vi "BCU参数读取-Auto.vi"(8 "CAN端口":u16(ring), 9 "设备索引号":u16(ring), 10 "CAN卡类型":u32(ring)=21, 11 "Myindex":dbl=1.0) -> (3 "成功":bool)   [LabVIEW 2013] (continued)
                                shift-right: [w3929] -> w3923
                                shift-left: string[] [] -> [w3931]
                                i -> [w3927]
                                w3936 = 8 ("索引")
                                w3940 = 2 ("y")
                                n2325 = Multiply(x=w3927, y=w3940) -> (x*y=w3941:i32)
                                n2326 = Array Subset(array=w3942, index=w3941, length=w3940) -> (w3939:u8[])
                                n2327 = Index Array(array=w3939) -> (element #1=w3938:u8, element #2=w3937:u8)  [unwired: 2 in]
                                n2328 = call "二进制解析-8.6.vi"("索引"=w3936, "数值"=w3938) -> ("低位子数组"=w3935:i32[])  [unwired: 1 in, 2 out]
                                n2329 = call "二进制解析-8.6.vi"("索引"=w3936, "数值"=w3937) -> ("低位子数组"=w3934:i32[])  [unwired: 1 in, 2 out]
                                n2330 = Insert Into Array(array=w3935, new element=w3934) -> (w3933:i32[])  [unwired: 1 in]
                                n2331 = case shown="1" w3927 {
                                tunnel: [4 6] -> w3928
                                frame 0, Default {
                                }
                                frame 1 {
                                }
                                }
                                n2332 = Reverse 1D Array(array=w3933) -> (reversed array=w3932:i32[])
                                n2333 = for {
                                N: w3928 -> [_]
                                tunnel: w3932 -> [w3949] mode=indexing
                                tunnel: [w3945] -> w3930 mode=indexing
                                n2334 = Equal To 0?(x=w3949) -> (x = 0?=w3948:bool)
                                n2335 = Select(t="无", s=w3948, f="故障") -> (s? t:f=w3945:string)
                                }
                                n2336 = Insert Into Array(array=w3931, new element=w3930) -> (w3929:string[])  [unwired: 1 in]
                              }
                              n2337 = call "详细故障分解.vi"("名称"=string[] ["超时(pre-chg)", "后端开路(pre-chg)", "后端短路(pre-chg)", "预充电回路断开(pre-chg)", "正级继电器驱动故障(relay_driver)", "负级继电器驱动故障(relay_driver)", "预充电继电器驱动故障(relay_driver)", "充电继电器驱动故障(relay_driver)", "风机继电器驱动故障(relay_driver)", "加热继电器驱动故障(relay_driver)"], "故障输入口"=w3923) -> ("输出数组"=w3921:string[][])  [unwired: 1 in, 2 out]
                              n2338 = local write "电池故障"(w3921) -> ()
                            }
                          }
                        }
                        frame True {
                          n2339 = Index Array(array=w3953, index #1=0 ("索引"), index #2=1 ("索引")) -> (element #1=w3956:u8, element #2=w3957:u8)
                          n2340 = Join Numbers(hi=w3956, lo=w3957) -> ((hi.lo)=w3955:u16)
                          n2341 = Number To Hexadecimal String(2:w3955) -> (0:w3954:string)  [unwired: 1 out]
                          n2342 = Concatenate Strings("读取错误，代码： " ("字符串"), "0x" ("字符串"), w3954) -> (w3952:string)
                          n2343 = One Button Dialog(message=w3952, button name ("OK")="是" ("按钮名称（“确定”）")) -> ()  [unwired: 1 out]
                        }
                      }
                      n2344 = local write "消除"(FALSE ("消除")) -> ()
                      n2345 = global write "EV05全局变量1.vi" "流控帧 2"(FALSE ("流控帧 2")) -> ()
                      n2346 = local write "控制1"(FALSE ("控制1")) -> ()
                      n2347 = global write "EV05全局变量1.vi" "写入超时"(TRUE ("写入超时")) -> ()
                    }
                  }
                }
              }
            }
          }
        }
      }
      frame Error {
      }
    }
  }
  n2348 = disable-structure shown="启用" {
    disable-tunnel: w32 -> [w3968 _]
    disable-tunnel: w24 -> [w3963 _]
    disable-tunnel: w21 -> [w3962 _]
    disable-tunnel: w1 -> [w3961 _]
    frame Disabled {
      n2349 = while {
        tunnel: w3968 -> [w3977]
        tunnel: w3961 -> [w3976]
        tunnel: [w3975] -> w3967
        tunnel: [w3974] -> w3966
        tunnel: w3963 -> [_]
        tunnel: w3962 -> [_]
        stop <- w3973 stop-if-true
        n2350 = event shown="[49] \"全部读取\": 值改变" {
          selector: _ -> [_ _ _ _ _ _ _ _ _ _ _ _ _ _ _ _ _ _ _ _ _ _ _ _ _ _ _ _ _ _ _ _ _ _ _ _ _ _ _ _ _ _ _ _ _ _ _ _ _ _ _ _ _]
          dyn-events: _ -> [_ _ _ _ _ _ _ _ _ _ _ _ _ _ _ _ _ _ _ _ _ _ _ _ _ _ _ _ _ _ _ _ _ _ _ _ _ _ _ _ _ _ _ _ _ _ _ _ _ _ _ _ _]
          timeout: 200 -> [_ _ _ _ _ _ _ _ _ _ _ _ _ _ _ _ _ _ _ _ _ _ _ _ _ _ _ _ _ _ _ _ _ _ _ _ _ _ _ _ _ _ _ _ _ _ _ _ _ _ _ _ _]
          tunnel: [_ w3980 w4020 _ _ _ _ _ _ _ _ _ _ _ _ _ _ _ _ _ _ _ _ _ _ _ _ _ _ _ _ _ _ _ _ _ _ _ _ _ _ _ _ _ _ _ _ _ _ _ _ _ _] -> w3972
          tunnel: w3977 -> [w3979 w3983 w4019 _ w4060 w4071 w4082 w4093 w4098 w4109 w4120 w4131 w4142 w4153 w4170 w4181 w4197 w4735 w5157 w5182 w5210 w5313 w5386 w5398 w5408 w5454 _ _ w5504 w5571 w5638 w5705 w5772 w5839 w5906 w5974 w6042 w6109 w6176 w6246 w6257 w6296 w6318 w6358 w6380 w6418 w6478 w6513 w6549 w6582 w6651 w6684 w6717]
          tunnel: w3976 -> [w3978 w3982 w4018 _ w4059 w4070 w4081 w4092 w4097 w4108 w4119 w4130 w4141 w4152 w4169 w4180 w4196 w4734 w5156 w5181 w5209 w5312 w5384 w5396 w5407 w5453 _ _ w5503 w5570 w5637 w5704 w5771 w5838 w5905 w5973 w6041 w6108 w6175 w6244 w6256 w6295 w6317 w6357 w6379 w6417 w6477 w6512 w6548 w6581 w6650 w6683 w6716]
          tunnel: [w3979 w3983 w4019 _ w4060 w4071 w4082 w4093 w4098 w4109 w4120 w4131 w4142 w4153 w4170 w4181 w4197 w4735 w5157 w5182 w5210 w5313 w5385 w5397 w5408 w5454 _ _ w5504 w5571 w5638 w5705 w5772 w5839 w5906 w5974 w6042 w6109 w6176 w6245 w6255 w6294 w6316 w6356 w6378 w6418 w6476 w6511 w6547 w6580 w6649 w6682 w6715] -> w3975
          tunnel: [w3978 w3982 w4018 _ w4059 w4070 w4081 w4092 w4097 w4108 w4119 w4130 w4141 w4152 w4169 w4180 w4196 w4734 w5156 w5181 w5209 w5312 w5383 w5395 w5407 w5453 _ _ w5503 w5570 w5637 w5704 w5771 w5838 w5905 w5973 w6041 w6108 w6175 w6243 w6254 w6293 w6315 w6355 w6377 w6417 w6475 w6510 w6546 w6579 w6648 w6681 w6714] -> w3974
          tunnel: [_ _ _ _ _ _ _ _ _ _ _ _ _ _ _ _ _ _ _ _ _ _ _ _ _ _ _ _ _ _ _ _ _ _ _ _ _ _ _ _ w6254 w6293 w6315 w6355 w6377 _ w6475 w6510 w6546 w6579 w6648 w6681 w6714] -> w3971
          event Timeout {
            n2351 = event-data() -> ()  [unwired: 3 out]
          }
          event "停止": Value Change {
            n2352 = event-data() -> ("NewVal"=w3981:bool)  [unwired: 5 out]
            n2353 = stacked-sequence {
              tunnel: w3981 -> [w4000 _]
              tunnel: [w4000 _] -> w3980
              frame #0 {
                n2354 = global read "配置文件全局.vi" "诊断标定读取地址"() -> (w3984:path)
                n2355 = call <vilib>:"Application Directory.vi"() -> ("Application Directory"=w3994:path)
                n2356 = property class="VI"("FP.State"=T29."Hidden" ("前面板窗口:状态")) -> (reference out=w3996:refnum<vi>, error out=w3995:errorcluster)  [unwired: 2 in]
                n2357 = Build Path(base path=w3994, name or relative path="config.ini" ("名称或相对路径")) -> (appended path=w3992:path)
                n2358 = call <vilib>:"Open Config Data.vi"("configuration file path"=w3992) -> ("error out"=w3989:errorcluster, "refnum"=w3991:T25)  [unwired: 8 in, 1 out]
                n2359 = local write "停止"(TRUE ("停止")) -> ()
                n2360 = property class="VI"(reference=w3996, error in=w3995, "Front Panel.Open"=FALSE ("前面板窗口:打开")) -> ()  [unwired: 2 out]
                n2361 = call-poly <vilib>:"Write Key.vi"("section"="总信息", "error in (no error)"=w3989, "value"=w3984, "key"="诊断标定读取地址" ("section"), "refnum"=w3991) -> ("error out"=w3988:errorcluster, "refnum out"=w3987:T25)  [unwired: 4 in, 1 out]
                n2362 = call <vilib>:"Close Config Data.vi"("error in (no error)"=w3988, "refnum"=w3987) -> ("error out"=w3986:errorcluster)  [unwired: 8 in, 1 out]
                n2363 = call <vilib>:"Clear Errors.vi"("error in (no error)"=w3986) -> ()  [unwired: 6 in, 1 out]
              }
              frame #1 {
                n2364 = disable-structure shown="禁用" {
                  frame Disabled {
                    n2365 = local read "设备索引号"() -> (w4006:u16)
                    n2366 = local read "CAN卡类型"() -> (w4007:u32)
                    n2367 = local read "CAN端口"() -> (w4005:u16)
                    n2368 = Build Array(7) -> (w4002:i32[])
                    n2369 = call "transmit-8.6.vi"("can卡类型"=w4007, "设备索引号"=w4006, "CAN端口"=w4005, "ID"=418398080, "SendType"=u8 0, "Data"=w4002) -> ()  [unwired: 3 in, 11 out]
                  }
                  frame Enabled {
                    w4014 = u8 0 items=["Normal", "Listen Only"] ("工作方式")
                    w4013 = u8 1 items=["Dual Filter", "Single Filter"] ("滤波方式")
                    n2370 = local read "设备索引号"() -> (w4009:u16)
                    n2371 = local read "CAN卡类型"() -> (w4008:u32)
                    n2372 = local read "CAN端口"() -> (w4010:u16)
                    n2373 = call "CAN_Init-8.6.vi"("CAN卡类型"=w4008, "设备索引号"=w4009, "CAN端口"=w4010, "操作类型"=enum16{"初始化CAN", "关闭CAN"}."初始化CAN", "滤波方式"=w4013, "Accept Code"=u32 0, "簇"=T21 {"打开CAN"=FALSE, "初始化CAN"=TRUE, "开始CAN"=TRUE, "重启"=FALSE, "关闭CAN"=FALSE}, "Mask Code"=u32 4294967295 ("Accept Code"), "工作方式"=w4014, "是否滤波"=FALSE) -> ()  [unwired: 4 in, 6 out]
                  }
                }
              }
            }
          }
          event Panel Close? {
            n2374 = event-data() -> ()  [unwired: 5 out]
            n2375 = stacked-sequence {
              tunnel: [w4033 _] -> w4020
              frame #0 {
                w4033 = TRUE ("前面板窗口:打开")
                n2376 = global read "配置文件全局.vi" "诊断标定读取地址"() -> (w4022:path)
                n2377 = call <vilib>:"Application Directory.vi"() -> ("Application Directory"=w4032:path)
                n2378 = property class="VI"("FP.State"=T29."Hidden" ("前面板窗口:状态")) -> (reference out=w4035:refnum<vi>, error out=w4034:errorcluster)  [unwired: 2 in]
                n2379 = Build Path(base path=w4032, name or relative path="config.ini" ("名称或相对路径")) -> (appended path=w4030:path)
                n2380 = call <vilib>:"Open Config Data.vi"("configuration file path"=w4030) -> ("error out"=w4027:errorcluster, "refnum"=w4029:T25)  [unwired: 8 in, 1 out]
                n2381 = property class="VI"(reference=w4035, error in=w4034, "Front Panel.Open"=FALSE ("前面板窗口:打开")) -> ()  [unwired: 2 out]
                n2382 = call-poly <vilib>:"Write Key.vi"("section"="总信息", "error in (no error)"=w4027, "value"=w4022, "key"="诊断标定读取地址" ("section"), "refnum"=w4029) -> ("error out"=w4026:errorcluster, "refnum out"=w4025:T25)  [unwired: 4 in, 1 out]
                n2383 = call <vilib>:"Close Config Data.vi"("error in (no error)"=w4026, "refnum"=w4025) -> ("error out"=w4024:errorcluster)  [unwired: 8 in, 1 out]
                n2384 = call <vilib>:"Clear Errors.vi"("error in (no error)"=w4024) -> ()  [unwired: 6 in, 1 out]
                n2385 = local write "强制终止读写标记"(TRUE ("强制终止读写标记")) -> ()
                n2386 = local write "停止"(w4033) -> ()
              }
              frame #1 {
                w4041 = u8 0 items=["Normal", "Listen Only"] ("工作方式")
                w4042 = u8 1 items=["Dual Filter", "Single Filter"] ("滤波方式")
                n2387 = local read "设备索引号"() -> (w4046:u16)
                n2388 = local read "CAN卡类型"() -> (w4047:u32)
                n2389 = local read "CAN端口"() -> (w4045:u16)
                n2390 = call "CAN_Init-8.6.vi"("CAN卡类型"=w4047, "设备索引号"=w4046, "CAN端口"=w4045, "操作类型"=enum16{"初始化CAN", "关闭CAN"}."初始化CAN", "滤波方式"=w4042, "Accept Code"=u32 0, "簇"=T21 {"打开CAN"=FALSE, "初始化CAN"=TRUE, "开始CAN"=TRUE, "重启"=FALSE, "关闭CAN"=FALSE}, "Mask Code"=u32 4294967295 ("Accept Code"), "工作方式"=w4041, "是否滤波"=FALSE) -> ()  [unwired: 4 in, 6 out]
              }
            }
            n2391 = event-data("Discard?"=w4020) -> ()  [unwired: 1 in, 1 out]
          }
          event "终止读写按钮": Value Change {
            n2392 = event-data() -> ("NewVal"=w4048:bool)  [unwired: 6 out]
            n2393 = case shown="真" w4048 {
              frame False {
              }
              frame True {
                n2394 = local write "强制终止读写标记"(TRUE ("强制终止读写标记")) -> ()
              }
            }
          }
          event "1": Value Change {
            w4057 = FALSE ("1")
            n2395 = event-data() -> ()  [unwired: 7 out]
            n2396 = local write "主板2"(T8."项目信息" ("主从板")) -> ()
            n2397 = Not(x=w4057) -> (.not. x?=w4056:bool)
            n2398 = local write "1"(w4056) -> ()
            n2399 = local write "1 2"(w4057) -> ()
            n2400 = local write "1 3"(w4057) -> ()
            n2401 = local write "1 4"(w4057) -> ()
            n2402 = local write "1 5"(w4057) -> ()
            n2403 = local write "1 11"(w4057) -> ()
            n2404 = global read "功能码全局.vi" "主板监控2"() -> (w4055:bool[])
            n2405 = Index Array(array=w4055, index=6 ("索引")) -> (element=w4050:bool)
            n2406 = Select(t=0, s=w4050, f=1) -> (s? t:f=w4051:i32)
            n2407 = property on="项目信息" class="Tbl (严格)"("Disabled"=w4051) -> ()  [unwired: 2 in, 2 out]
            n2408 = property on="电池实际容量(A)" class="DigNum (严格)"("Disabled"=w4051) -> ()  [unwired: 2 in, 2 out]
            n2409 = property on="使用者" class="DigNum (严格)"("Disabled"=w4051) -> ()  [unwired: 2 in, 2 out]
            n2410 = property on="SOH(%)" class="DigNum (严格)"("Disabled"=w4051) -> ()  [unwired: 2 in, 2 out]
            n2411 = property on="电池额定容量(A)" class="DigNum (严格)"("Disabled"=w4051) -> ()  [unwired: 2 in, 2 out]
            n2412 = property on="SOC(%)" class="DigNum (严格)"("Disabled"=w4051) -> ()  [unwired: 2 in, 2 out]
            n2413 = property on="项目信息2" class="Clust (严格)"("DisabledEnum"=w4051) -> ()  [unwired: 2 in, 2 out]
            n2414 = property on="系统时钟" class="Str"("Disabled"=w4051) -> ()  [unwired: 2 in, 2 out]
            n2415 = property on="配置文件版本" class="Str"("Disabled"=w4051) -> ()  [unwired: 2 in, 2 out]
            n2416 = property on="车架(牌)号" class="Str"("Disabled"=w4051) -> ()  [unwired: 2 in, 2 out]
            n2417 = property on="产品编号" class="Str"("Disabled"=w4051) -> ()  [unwired: 2 in, 2 out]
          }
          event "1 2": Value Change {
            w4068 = FALSE ("1")
            n2418 = event-data() -> ()  [unwired: 7 out]
            n2419 = local write "主板2"(T8."一级故障阀值" ("主从板")) -> ()
            n2420 = Not(x=w4068) -> (.not. x?=w4067:bool)
            n2421 = local write "1"(w4068) -> ()
            n2422 = local write "1 2"(w4067) -> ()
            n2423 = local write "1 3"(w4068) -> ()
            n2424 = local write "1 4"(w4068) -> ()
            n2425 = local write "1 5"(w4068) -> ()
            n2426 = local write "1 11"(w4068) -> ()
            n2427 = global read "功能码全局.vi" "主板监控2"() -> (w4066:bool[])
            n2428 = Index Array(array=w4066, index=6 ("索引")) -> (element=w4061:bool)
            n2429 = Select(t=0, s=w4061, f=1) -> (s? t:f=w4064:i32)
            n2430 = property on="一级故障" class="Clust (严格)"("DisabledEnum"=w4064) -> ()  [unwired: 2 in, 2 out]
          }
          event "1 3": Value Change {
            w4079 = FALSE ("1")
            n2431 = event-data() -> ()  [unwired: 7 out]
            n2432 = local write "主板2"(T8."二级故障阀值" ("主从板")) -> ()
            n2433 = Not(x=w4079) -> (.not. x?=w4078:bool)
            n2434 = local write "1"(w4079) -> ()
            n2435 = local write "1 2"(w4079) -> ()
            n2436 = local write "1 3"(w4078) -> ()
            n2437 = local write "1 4"(w4079) -> ()
            n2438 = local write "1 5"(w4079) -> ()
            n2439 = local write "1 11"(w4079) -> ()
            n2440 = global read "功能码全局.vi" "主板监控2"() -> (w4077:bool[])
            n2441 = Index Array(array=w4077, index=6 ("索引")) -> (element=w4073:bool)
            n2442 = Select(t=0, s=w4073, f=1) -> (s? t:f=w4072:i32)
            n2443 = property on="一级故障 2" class="Clust (严格)"("DisabledEnum"=w4072) -> ()  [unwired: 2 in, 2 out]
          }
          event "1 4": Value Change {
            w4090 = FALSE ("1")
            n2444 = event-data() -> ()  [unwired: 7 out]
            n2445 = local write "主板2"(T8."三级故障阀值" ("主从板")) -> ()
            n2446 = Not(x=w4090) -> (.not. x?=w4089:bool)
            n2447 = local write "1"(w4090) -> ()
            n2448 = local write "1 2"(w4090) -> ()
            n2449 = local write "1 3"(w4090) -> ()
            n2450 = local write "1 4"(w4089) -> ()
            n2451 = local write "1 5"(w4090) -> ()
            n2452 = local write "1 11"(w4090) -> ()
            n2453 = global read "功能码全局.vi" "主板监控2"() -> (w4088:bool[])
            n2454 = Index Array(array=w4088, index=6 ("索引")) -> (element=w4083:bool)
            n2455 = Select(t=0, s=w4083, f=1) -> (s? t:f=w4086:i32)
            n2456 = property on="一级故障 3" class="Clust (严格)"("DisabledEnum"=w4086) -> ()  [unwired: 2 in, 2 out]
          }
          event "1 5": Value Change {
            w4095 = FALSE ("1")
            n2457 = event-data() -> ()  [unwired: 7 out]
            n2458 = local write "主板2"(T8."控制参数" ("主从板")) -> ()
            n2459 = Not(x=w4095) -> (.not. x?=w4094:bool)
            n2460 = local write "1"(w4095) -> ()
            n2461 = local write "1 2"(w4095) -> ()
            n2462 = local write "1 3"(w4095) -> ()
            n2463 = local write "1 4"(w4095) -> ()
            n2464 = local write "1 5"(w4094) -> ()
            n2465 = local write "1 11"(w4095) -> ()
            n2466 = disable-structure shown="禁用" {
              frame Disabled {
                n2467 = global read "功能码全局.vi" "主板监控2"() -> (w4102:bool[])
                n2468 = Index Array(array=w4102, index=6 ("索引")) -> (element=w4100:bool)
                n2469 = Select(t=0, s=w4100, f=1) -> (s? t:f=w4099:i32)
                n2470 = property on="风机开启温度" class="DigNum (严格)"("Disabled"=w4099) -> ()  [unwired: 2 in, 2 out]
                n2471 = property on="风机关闭温度" class="DigNum (严格)"("Disabled"=w4099) -> ()  [unwired: 2 in, 2 out]
                n2472 = property on="加热开启温度" class="DigNum (严格)"("Disabled"=w4099) -> ()  [unwired: 2 in, 2 out]
                n2473 = property on="加热关闭温度" class="DigNum (严格)"("Disabled"=w4099) -> ()  [unwired: 2 in, 2 out]
                n2474 = property on="风机开启温差" class="DigNum (严格)"("Disabled"=w4099) -> ()  [unwired: 2 in, 2 out]
                n2475 = property on="风机关闭温差" class="DigNum (严格)"("Disabled"=w4099) -> ()  [unwired: 2 in, 2 out]
                n2476 = property on="加热控制参数" class="Clust (严格)"("DisabledEnum"=w4099) -> ()  [unwired: 2 in, 2 out]
                n2477 = property on="最大允许总电压" class="DigNum (严格)"("Disabled"=w4099) -> ()  [unwired: 2 in, 2 out]
                n2478 = property on="最大允许充电温度" class="DigNum (严格)"("Disabled"=w4099) -> ()  [unwired: 2 in, 2 out]
                n2479 = property on="最小允许充电温度" class="DigNum (严格)"("Disabled"=w4099) -> ()  [unwired: 2 in, 2 out]
                n2480 = property on="电流步长" class="DigNum (严格)"("Disabled"=w4099) -> ()  [unwired: 2 in, 2 out]
                n2481 = property on="最大允许单体电压" class="DigNum (严格)"("Disabled"=w4099) -> ()  [unwired: 2 in, 2 out]
                n2482 = property on="最小允许单体电压" class="DigNum (严格)"("Disabled"=w4099) -> ()  [unwired: 2 in, 2 out]
                n2483 = property on="最大允许充电电流" class="DigNum (严格)"("Disabled"=w4099) -> ()  [unwired: 2 in, 2 out]
                n2484 = property on="最小允许充电电流" class="DigNum (严格)"("Disabled"=w4099) -> ()  [unwired: 2 in, 2 out]
              }
              frame Enabled {
              }
            }
          }
          event "1 11": Value Change {
            w4106 = FALSE ("1")
            n2485 = event-data() -> ()  [unwired: 7 out]
            n2486 = local write "主板2"(T8."电池信息" ("主从板")) -> ()
            n2487 = Not(x=w4106) -> (.not. x?=w4105:bool)
            n2488 = local write "1"(w4106) -> ()
            n2489 = local write "1 2"(w4106) -> ()
            n2490 = local write "1 3"(w4106) -> ()
            n2491 = local write "1 4"(w4106) -> ()
            n2492 = local write "1 5"(w4106) -> ()
            n2493 = local write "1 11"(w4105) -> ()
            n2494 = disable-structure shown="禁用" {
              frame Disabled {
                n2495 = global read "功能码全局.vi" "主板监控2"() -> (w4112:bool[])
                n2496 = Index Array(array=w4112, index=6 ("索引")) -> (element=w4110:bool)
                n2497 = Select(t=0, s=w4110, f=1) -> (s? t:f=w4113:i32)
                n2498 = property on="电池串联" class="DigNum (严格)"("Disabled"=w4113) -> ()  [unwired: 2 in, 2 out]
                n2499 = property on="电池并联" class="DigNum (严格)"("Disabled"=w4113) -> ()  [unwired: 2 in, 2 out]
                n2500 = property on="电池包额定容量" class="DigNum (严格)"("Disabled"=w4113) -> ()  [unwired: 2 in, 2 out]
                n2501 = property on="电池包额定能量(kWh)" class="DigNum (严格)"("Disabled"=w4113) -> ()  [unwired: 2 in, 2 out]
                n2502 = property on="电池包额定总电压" class="DigNum (严格)"("Disabled"=w4113) -> ()  [unwired: 2 in, 2 out]
                n2503 = property on="实际容量" class="DigNum (严格)"("Disabled"=w4113) -> ()  [unwired: 2 in, 2 out]
                n2504 = property on="电池包组号" class="Str"("Disabled"=w4113) -> ()  [unwired: 2 in, 2 out]
                n2505 = property on="电池生产日期" class="Str"("Disabled"=w4113) -> ()  [unwired: 2 in, 2 out]
                n2506 = property on="电池厂家" class="Str"("Disabled"=w4113) -> ()  [unwired: 2 in, 2 out]
                n2507 = property on="电池类型" class="Str"("Disabled"=w4113) -> ()  [unwired: 2 in, 2 out]
                n2508 = property on="累计充电总安时" class="DigNum (严格)"("Disabled"=w4113) -> ()  [unwired: 2 in, 2 out]
                n2509 = property on="累计放电总安时" class="DigNum (严格)"("Disabled"=w4113) -> ()  [unwired: 2 in, 2 out]
                n2510 = property on="电池放空次数" class="DigNum (严格)"("Disabled"=w4113) -> ()  [unwired: 2 in, 2 out]
                n2511 = property on="电池充满次数" class="DigNum (严格)"("Disabled"=w4113) -> ()  [unwired: 2 in, 2 out]
                n2512 = property on="电池充电次数" class="DigNum (严格)"("Disabled"=w4113) -> ()  [unwired: 2 in, 2 out]
                n2513 = property on="电池信息" class="Clust (严格)"("DisabledEnum"=w4113) -> ()  [unwired: 2 in, 2 out]
              }
              frame Enabled {
              }
            }
          }
          event "1 6": Value Change {
            w4117 = FALSE ("1 6")
            n2514 = event-data() -> ()  [unwired: 7 out]
            n2515 = Not(x=w4117) -> (.not. x?=w4116:bool)
            n2516 = local write "1 6"(w4116) -> ()
            n2517 = local write "1 7"(w4117) -> ()
            n2518 = local write "1 8"(w4117) -> ()
            n2519 = local write "1 9"(w4117) -> ()
            n2520 = local write "1 10"(w4117) -> ()
            n2521 = local write "等级 2"(T19."从板信息" ("等级 2")) -> ()
            n2522 = disable-structure shown="禁用" {
              frame Disabled {
                n2523 = global read "功能码全局.vi" "主板监控2"() -> (w4123:bool[])
                n2524 = Index Array(array=w4123, index=6 ("索引")) -> (element=w4121:bool)
                n2525 = Select(t=0, s=w4121, f=1) -> (s? t:f=w4124:i32)
                n2526 = property on="项目信息 2" class="Tbl (严格)"("Disabled"=w4124) -> ()  [unwired: 2 in, 2 out]
                n2527 = property on="加热控制参数" class="Clust (严格)"("Disabled"=w4124) -> ()  [unwired: 2 in, 2 out]
              }
              frame Enabled {
              }
            }
          }
          event "1 7": Value Change {
            w4128 = FALSE ("1 6")
            n2528 = event-data() -> ()  [unwired: 7 out]
            n2529 = disable-structure shown="禁用" {
              frame Disabled {
                n2530 = global read "功能码全局.vi" "主板监控2"() -> (w4137:bool[])
                n2531 = Index Array(array=w4137, index=6 ("索引")) -> (element=w4132:bool)
                n2532 = Select(t=0, s=w4132, f=1) -> (s? t:f=w4133:i32)
                n2533 = property on="一级故障 6" class="Clust (严格)"("DisabledEnum"=w4133) -> ()  [unwired: 2 in, 2 out]
              }
              frame Enabled {
              }
            }
            n2534 = local write "等级 2"(T19."一级故障阀值" ("等级 2")) -> ()
            n2535 = Not(x=w4128) -> (.not. x?=w4127:bool)
            n2536 = local write "1 6"(w4128) -> ()
            n2537 = local write "1 7"(w4127) -> ()
            n2538 = local write "1 8"(w4128) -> ()
            n2539 = local write "1 9"(w4128) -> ()
            n2540 = local write "1 10"(w4128) -> ()
          }
          event "1 8": Value Change {
            w4139 = FALSE ("1 6")
            n2541 = event-data() -> ()  [unwired: 7 out]
            n2542 = disable-structure shown="禁用" {
              frame Disabled {
                n2543 = global read "功能码全局.vi" "主板监控2"() -> (w4148:bool[])
                n2544 = Index Array(array=w4148, index=6 ("索引")) -> (element=w4143:bool)
                n2545 = Select(t=0, s=w4143, f=1) -> (s? t:f=w4144:i32)
                n2546 = property on="一级故障 7" class="Clust (严格)"("DisabledEnum"=w4144) -> ()  [unwired: 2 in, 2 out]
              }
              frame Enabled {
              }
            }
            n2547 = local write "等级 2"(T19."二级故障阀值" ("等级 2")) -> ()
            n2548 = Not(x=w4139) -> (.not. x?=w4138:bool)
            n2549 = local write "1 6"(w4139) -> ()
            n2550 = local write "1 7"(w4139) -> ()
            n2551 = local write "1 8"(w4138) -> ()
            n2552 = local write "1 9"(w4139) -> ()
            n2553 = local write "1 10"(w4139) -> ()
          }
          event "1 9": Value Change {
            w4150 = FALSE ("1 6")
            n2554 = event-data() -> ()  [unwired: 7 out]
            n2555 = disable-structure shown="禁用" {
              frame Disabled {
                n2556 = global read "功能码全局.vi" "主板监控2"() -> (w4159:bool[])
                n2557 = Index Array(array=w4159, index=6 ("索引")) -> (element=w4154:bool)
                n2558 = Select(t=0, s=w4154, f=1) -> (s? t:f=w4155:i32)
                n2559 = property on="一级故障 8" class="Clust (严格)"("DisabledEnum"=w4155) -> ()  [unwired: 2 in, 2 out]
              }
              frame Enabled {
              }
            }
            n2560 = local write "等级 2"(T19."三级故障阀值" ("等级 2")) -> ()
            n2561 = Not(x=w4150) -> (.not. x?=w4149:bool)
            n2562 = local write "1 6"(w4150) -> ()
            n2563 = local write "1 7"(w4150) -> ()
            n2564 = local write "1 8"(w4150) -> ()
            n2565 = local write "1 9"(w4149) -> ()
            n2566 = local write "1 10"(w4150) -> ()
          }
          event "1 10": Value Change {
            w4167 = FALSE ("1 6")
            n2567 = event-data() -> ()  [unwired: 7 out]
            n2568 = global read "功能码全局.vi" "主板监控2"() -> (w4165:bool[])
            n2569 = Index Array(array=w4165, index=6 ("索引")) -> (element=w4160:bool)
            n2570 = Select(t=0, s=w4160, f=1) -> (s? t:f=w4161:i32)
            n2571 = local write "等级 2"(T19."快换参数" ("等级 2")) -> ()
            n2572 = property on="电池组信息" class="Clust (严格)"("Disabled"=w4161) -> ()  [unwired: 2 in, 2 out]
            n2573 = Not(x=w4167) -> (.not. x?=w4166:bool)
            n2574 = local write "1 6"(w4167) -> ()
            n2575 = local write "1 7"(w4167) -> ()
            n2576 = local write "1 8"(w4167) -> ()
            n2577 = local write "1 9"(w4167) -> ()
            n2578 = local write "1 10"(w4166) -> ()
          }
          event "1 12": Value Change {
            w4172 = FALSE ("1 6")
            n2579 = event-data() -> ()  [unwired: 7 out]
            n2580 = global read "功能码全局.vi" "主板监控2"() -> (w4179:bool[])
            n2581 = Index Array(array=w4179, index=6 ("索引")) -> (element=w4175:bool)
            n2582 = Select(t=0, s=w4175, f=1) -> (s? t:f=w4171:i32)
            n2583 = local write "等级 2"(T14."均衡参数" ("等级 2")) -> ()
            n2584 = property on="均衡参数" class="Clust (严格)"("DisabledEnum"=w4171) -> ()  [unwired: 2 in, 2 out]
            n2585 = Not(x=w4172) -> (.not. x?=w4173:bool)
            n2586 = local write "1 12"(w4173) -> ()
            n2587 = local write "1 6"(w4172) -> ()
            n2588 = local write "1 7"(w4172) -> ()
            n2589 = local write "1 8"(w4172) -> ()
            n2590 = local write "1 9"(w4172) -> ()
            n2591 = local write "1 10"(w4172) -> ()
          }
          event "主板选项": Mouse Down {
            n2592 = event-data() -> ("CtlRef"=w4195:refnum<vi>)  [unwired: 8 out]
            n2593 = global read "功能码全局.vi" "主板监控2"() -> (w4184:bool[])
            n2594 = property class="Tree (严格)"(reference=w4195) -> ("Value"=w4187:string)  [unwired: 1 in, 2 out]
            n2595 = Index Array(array=w4184, index=6 ("索引")) -> (element=w4182:bool)
            n2596 = case shown="\"二维码\"" w4187 {
              tunnel: [T8."项目信息" ("主从板") T8."项目信息" ("主从板") T8."项目信息" ("主从板") T8."项目信息" ("主从板") T8."项目信息" ("主从板") T8."项目信息" ("主从板") T8."项目信息" ("主从板") T8."项目信息" ("主从板") T8."项目信息" ("主从板") T8."项目信息" ("主从板") T8."项目信息" ("主从板") T8."项目信息" ("主从板") T8."项目信息" ("主从板") T8."项目信息" ("主从板") T8."项目信息" ("主从板") T8."项目信息" ("主从板") T8."二级故障阀值" ("主从板") T8."三级故障阀值" ("主从板") T8."一级故障阀值" ("主从板") T8."控制参数" ("主从板") T8."控制参数" ("主从板") T8."电池信息" ("主从板") T8."电池信息" ("主从板") T8."电池信息" ("主从板") T8."电池信息" ("主从板") T8."电池信息" ("主从板") T8."项目信息" ("主从板")] -> w4194
              tunnel: [w4205 w4212 w4227 w4242 w4259 w4299 w4333 w4380 w4418 w4468 w4503 w4517 w4532 w4547 w4562 w4576 w4589 w4603 w4616 w4630 w4644 w4657 w4671 w4685 w4699 w4713 w4717] -> w4193
              tunnel: [w4206 w4213 w4228 w4243 w4260 w4300 w4334 w4381 w4419 w4469 w4504 w4518 w4533 w4548 w4563 w4577 w4589 w4603 w4615 w4630 w4644 w4657 w4671 w4685 w4699 w4713 w4718] -> w4192
              tunnel: [w4206 w4213 w4228 w4243 w4260 w4300 w4334 w4381 w4419 w4469 w4504 w4518 w4533 w4548 w4563 w4577 w4590 w4603 w4616 w4630 w4644 w4657 w4671 w4685 w4699 w4713 w4718] -> w4191
              tunnel: [w4206 w4213 w4228 w4243 w4260 w4300 w4334 w4381 w4419 w4469 w4504 w4518 w4533 w4548 w4563 w4577 w4589 w4602 w4616 w4630 w4644 w4657 w4671 w4685 w4699 w4713 w4718] -> w4190
              tunnel: [w4206 w4213 w4228 w4243 w4260 w4300 w4334 w4381 w4419 w4469 w4504 w4518 w4533 w4548 w4563 w4577 w4589 w4603 w4616 w4629 w4643 w4657 w4671 w4685 w4699 w4713 w4718] -> w4189
              tunnel: [w4206 w4213 w4228 w4243 w4260 w4300 w4334 w4381 w4419 w4469 w4504 w4518 w4533 w4548 w4563 w4577 w4589 w4603 w4616 w4630 w4644 w4656 w4670 w4684 w4698 w4712 w4718] -> w4188
              tunnel: [w4198 FALSE w4223 w4238 w4251 w4291 w4324 w4371 w4410 w4461 w4498 w4512 w4526 w4540 w4555 w4571 w4585 w4598 w4611 w4625 w4638 w4652 w4665 w4679 w4693 w4707 FALSE] -> w4186
              tunnel: [w4198 TRUE w4220 w4235 w4250 w4290 w4325 w4372 w4409 w4460 w4497 w4511 w4525 w4541 w4556 w4570 w4584 w4597 w4610 w4624 w4637 w4651 w4664 w4678 w4692 w4706 FALSE] -> w4185
              tunnel: w4182 -> [w4203 _ w4217 w4232 w4247 w4286 w4321 w4368 w4406 w4458 w4494 w4508 w4522 w4537 w4552 w4567 w4581 w4594 w4607 w4621 w4634 w4648 w4661 w4675 w4689 w4703 _]
              frame "项目信息" {
                w4206 = FALSE
                n2597 = Select(t=0, s=w4203, f=1) -> (s? t:f=w4201:i32)
                n2598 = property on="项目信息" class="Tbl (严格)"("Disabled"=w4201) -> ()  [unwired: 2 in, 2 out]
                n2599 = property on="电池实际容量(A)" class="DigNum (严格)"("Disabled"=w4201) -> ()  [unwired: 2 in, 2 out]
                n2600 = property on="使用者" class="DigNum (严格)"("Disabled"=w4201) -> ()  [unwired: 2 in, 2 out]
                n2601 = property on="SOH(%)" class="DigNum (严格)"("Disabled"=w4201) -> ()  [unwired: 2 in, 2 out]
                n2602 = property on="从板个数" class="DigNum (严格)"("NumText.BGColor"=u32 6618880) -> ()  [unwired: 2 in, 2 out]
                n2603 = property on="电池额定容量(A)" class="DigNum (严格)"("Disabled"=w4201) -> ()  [unwired: 2 in, 2 out]
                n2604 = property on="SOC(%)" class="DigNum (严格)"("Disabled"=w4201) -> ()  [unwired: 2 in, 2 out]
                n2605 = property on="项目信息2" class="Clust (严格)"("DisabledEnum"=w4201) -> ()  [unwired: 2 in, 2 out]
                n2606 = property on="系统时钟" class="Str"("Disabled"=w4201) -> ()  [unwired: 2 in, 2 out]
                n2607 = property on="配置文件版本" class="Str"("Disabled"=w4201) -> ()  [unwired: 2 in, 2 out]
                n2608 = property on="车架(牌)号" class="Str"("Disabled"=w4201) -> ()  [unwired: 2 in, 2 out]
                n2609 = property on="产品编号" class="Str"("Disabled"=w4201) -> ()  [unwired: 2 in, 2 out]
                n2610 = local read "项目信息结果"() -> (w4199:bool)
                n2611 = Not(x=w4199) -> (.not. x?=w4198:bool)
                n2612 = Not(x=w4206) -> (.not. x?=w4205:bool)
              }
              frame "校正时钟" {
                w4209 = 2
                w4213 = FALSE
                n2613 = property on="从板个数" class="DigNum (严格)"("NumText.BGColor"=u32 13816530) -> ()  [unwired: 2 in, 2 out]
                n2614 = property on="项目信息" class="Tbl (严格)"("Disabled"=w4209) -> ()  [unwired: 2 in, 2 out]
                n2615 = property on="电池实际容量(A)" class="DigNum (严格)"("Disabled"=w4209) -> ()  [unwired: 2 in, 2 out]
                n2616 = property on="使用者" class="DigNum (严格)"("Disabled"=w4209) -> ()  [unwired: 2 in, 2 out]
                n2617 = property on="SOH(%)" class="DigNum (严格)"("Disabled"=w4209) -> ()  [unwired: 2 in, 2 out]
                n2618 = property on="电池额定容量(A)" class="DigNum (严格)"("Disabled"=w4209) -> ()  [unwired: 2 in, 2 out]
                n2619 = property on="SOC(%)" class="DigNum (严格)"("Disabled"=w4209) -> ()  [unwired: 2 in, 2 out]
                n2620 = property on="系统时钟" class="Str"("Disabled"=w4209) -> ()  [unwired: 2 in, 2 out]
                n2621 = property on="配置文件版本" class="Str"("Disabled"=w4209) -> ()  [unwired: 2 in, 2 out]
                n2622 = property on="车架(牌)号" class="Str"("Disabled"=w4209) -> ()  [unwired: 2 in, 2 out]
                n2623 = property on="项目信息2" class="Clust (严格)"("DisabledEnum"=w4209) -> ()  [unwired: 2 in, 2 out]
                n2624 = property on="产品编号" class="Str"("Disabled"=w4209) -> ()  [unwired: 2 in, 2 out]
                n2625 = Not(x=w4213) -> (.not. x?=w4212:bool)
              }
              frame "产品编号" {
                w4226 = 2
                w4228 = FALSE
                n2626 = property on="项目信息" class="Tbl (严格)"("Disabled"=w4226) -> ()  [unwired: 2 in, 2 out]
                n2627 = property on="电池实际容量(A)" class="DigNum (严格)"("Disabled"=w4226) -> ()  [unwired: 2 in, 2 out]
                n2628 = property on="使用者" class="DigNum (严格)"("Disabled"=w4226) -> ()  [unwired: 2 in, 2 out]
                n2629 = Select(t=0, s=w4217, f=1) -> (s? t:f=w4216:i32)
                n2630 = property on="SOH(%)" class="DigNum (严格)"("Disabled"=w4226) -> ()  [unwired: 2 in, 2 out]
                n2631 = property on="电池额定容量(A)" class="DigNum (严格)"("Disabled"=w4226) -> ()  [unwired: 2 in, 2 out]
                n2632 = property on="SOC(%)" class="DigNum (严格)"("Disabled"=w4226) -> ()  [unwired: 2 in, 2 out]
                n2633 = property on="产品编号" class="Str"("Disabled"=w4216) -> ()  [unwired: 2 in, 2 out]
                n2634 = property on="项目信息2" class="Clust (严格)"("DisabledEnum"=w4216) -> ()  [unwired: 2 in, 2 out]
                n2635 = property on="系统时钟" class="Str"("Disabled"=w4226) -> ()  [unwired: 2 in, 2 out]
                n2636 = property on="配置文件版本" class="Str"("Disabled"=w4226) -> ()  [unwired: 2 in, 2 out]
                n2637 = property on="车架(牌)号" class="Str"("Disabled"=w4226) -> ()  [unwired: 2 in, 2 out]
                n2638 = property on="从板个数" class="DigNum (严格)"("NumText.BGColor"=u32 13816530) -> ()  [unwired: 2 in, 2 out]
                n2639 = global read "功能码全局.vi" "主板项目信息5"() -> (w4224:bool[])
                n2640 = global read "功能码全局.vi" "主板项目信息6"() -> (w4221:bool[])
                n2641 = Index Array(array=w4224, index=0 ("索引")) -> (element=w4223:bool)
                n2642 = Index Array(array=w4221, index=1 ("索引")) -> (element=w4220:bool)
                n2643 = Not(x=w4228) -> (.not. x?=w4227:bool)
              }
              frame "二维码" {
                w4241 = 2
                w4243 = FALSE
                n2644 = property on="项目信息" class="Tbl (严格)"("Disabled"=w4241) -> ()  [unwired: 2 in, 2 out]
                n2645 = property on="电池实际容量(A)" class="DigNum (严格)"("Disabled"=w4241) -> ()  [unwired: 2 in, 2 out]
                n2646 = property on="使用者" class="DigNum (严格)"("Disabled"=w4241) -> ()  [unwired: 2 in, 2 out]
                n2647 = Select(t=0, s=w4232, f=1) -> (s? t:f=w4231:i32)
                n2648 = property on="SOH(%)" class="DigNum (严格)"("Disabled"=w4241) -> ()  [unwired: 2 in, 2 out]
                n2649 = property on="电池额定容量(A)" class="DigNum (严格)"("Disabled"=w4241) -> ()  [unwired: 2 in, 2 out]
                n2650 = property on="SOC(%)" class="DigNum (严格)"("Disabled"=w4241) -> ()  [unwired: 2 in, 2 out]
                n2651 = property on="产品编号" class="Str"("Disabled"=w4231) -> ()  [unwired: 2 in, 2 out]
                n2652 = property on="项目信息2" class="Clust (严格)"("DisabledEnum"=w4231) -> ()  [unwired: 2 in, 2 out]
                n2653 = property on="系统时钟" class="Str"("Disabled"=w4241) -> ()  [unwired: 2 in, 2 out]
                n2654 = property on="配置文件版本" class="Str"("Disabled"=w4241) -> ()  [unwired: 2 in, 2 out]
                n2655 = property on="车架(牌)号" class="Str"("Disabled"=w4241) -> ()  [unwired: 2 in, 2 out]
                n2656 = property on="从板个数" class="DigNum (严格)"("NumText.BGColor"=u32 13816530) -> ()  [unwired: 2 in, 2 out]
                n2657 = global read "功能码全局.vi" "主板项目信息5"() -> (w4239:bool[])
                n2658 = global read "功能码全局.vi" "主板项目信息6"() -> (w4236:bool[])
                n2659 = Index Array(array=w4239, index=0 ("索引")) -> (element=w4238:bool)
                n2660 = Index Array(array=w4236, index=1 ("索引")) -> (element=w4235:bool)
                n2661 = Not(x=w4243) -> (.not. x?=w4242:bool)
              }
              frame "电压个数" {
                w4258 = 2
                w4260 = FALSE
                n2662 = local read "从板个数"() -> (w4257:dbl)
                n2663 = property on="从板个数" class="DigNum (严格)"("NumText.BGColor"=u32 6618880) -> ()  [unwired: 2 in, 2 out]
                n2664 = property on="电池实际容量(A)" class="DigNum (严格)"("Disabled"=w4258) -> ()  [unwired: 2 in, 2 out]
                n2665 = property on="使用者" class="DigNum (严格)"("Disabled"=w4258) -> ()  [unwired: 2 in, 2 out]
                n2666 = property on="SOH(%)" class="DigNum (严格)"("Disabled"=w4258) -> ()  [unwired: 2 in, 2 out]
                n2667 = property on="电池额定容量(A)" class="DigNum (严格)"("Disabled"=w4258) -> ()  [unwired: 2 in, 2 out]
                n2668 = property on="SOC(%)" class="DigNum (严格)"("Disabled"=w4258) -> ()  [unwired: 2 in, 2 out]
                n2669 = property on="系统时钟" class="Str"("Disabled"=w4258) -> ()  [unwired: 2 in, 2 out]
                n2670 = property on="配置文件版本" class="Str"("Disabled"=w4258) -> ()  [unwired: 2 in, 2 out]
                n2671 = property on="车架(牌)号" class="Str"("Disabled"=w4258) -> ()  [unwired: 2 in, 2 out]
                n2672 = property on="产品编号" class="Str"("Disabled"=w4258) -> ()  [unwired: 2 in, 2 out]
                n2673 = Select(t=0, s=w4247, f=1) -> (s? t:f=w4246:i32)
                n2674 = control-ref of="项目信息"() -> (w4256:refnum<vi>)
                n2675 = stacked-sequence {
                  tunnel: w4257 -> [_ w4267 w4277]
                  tunnel: w4256 -> [w4262 w4266 w4278]
                  frame #0 {
                    w4263 = 0
                    n2676 = Bundle(w4263, w4263) -> (w4265:cluster{i32, i32})  [unwired: 1 out]
                    n2677 = property class="Tbl (严格)"(reference=w4262, "Index Values"=w4265) -> (error out=w4264:errorcluster)  [unwired: 1 in, 1 out]
                    n2678 = call <vilib>:"Clear Errors.vi"("error in (no error)"=w4264) -> ()  [unwired: 7 out]
                  }
                  frame #1 {
                    n2679 = for {
                      N: 10 -> [_]
                      tunnel: w4266 -> [w4276]
                      tunnel: w4267 -> [w4271]
                      i -> [w4270]
                      n2680 = Compound Arithmetic op=ADD(0.0 ("值"), w4271, w4270) -> (w4273:dbl)
                      n2681 = Bundle(w4273, 0) -> (w4275:cluster{dbl, i32})  [unwired: 1 out]
                      n2682 = property class="Tbl (严格)"(reference=w4276, "Active Cell"=w4275, "Cell BG Color"=u32 16448250) -> ()  [unwired: 1 in, 2 out]
                    }
                  }
                  frame #2 {
                    n2683 = for {
                      N: w4277 -> [_]
                      tunnel: w4278 -> [w4279]
                      i -> [w4280]
                      n2684 = Bundle(w4280, 0) -> (w4284:cluster{i32, i32})  [unwired: 1 out]
                      n2685 = property class="Tbl (严格)"(reference=w4279, "Active Cell"=w4284, "Cell BG Color"=u32 6618880) -> (error out=w4281:errorcluster)  [unwired: 1 in, 1 out]
                      n2686 = call <vilib>:"Clear Errors.vi"("error in (no error)"=w4281) -> ()  [unwired: 7 out]
                    }
                  }
                }
                n2687 = property on="项目信息" class="Tbl (严格)"("Disabled"=w4246) -> ()  [unwired: 2 in, 2 out]
                n2688 = global read "功能码全局.vi" "主板项目信息5"() -> (w4254:bool[])
                n2689 = global read "功能码全局.vi" "主板项目信息6"() -> (w4252:bool[])
                n2690 = Index Array(array=w4254, index=1 ("索引")) -> (element=w4251:bool)
                n2691 = Index Array(array=w4252, index=2 ("索引")) -> (element=w4250:bool)
                n2692 = Not(x=w4260) -> (.not. x?=w4259:bool)
              }
              frame "通道电压数" {
                w4298 = 2
                w4300 = FALSE
                n2693 = property on="从板个数" class="DigNum (严格)"("NumText.BGColor"=u32 13816530) -> ()  [unwired: 2 in, 2 out]
                n2694 = property on="电池实际容量(A)" class="DigNum (严格)"("Disabled"=w4298) -> ()  [unwired: 2 in, 2 out]
                n2695 = property on="使用者" class="DigNum (严格)"("Disabled"=w4298) -> ()  [unwired: 2 in, 2 out]
                n2696 = property on="SOH(%)" class="DigNum (严格)"("Disabled"=w4298) -> ()  [unwired: 2 in, 2 out]
                n2697 = property on="电池额定容量(A)" class="DigNum (严格)"("Disabled"=w4298) -> ()  [unwired: 2 in, 2 out]
                n2698 = property on="SOC(%)" class="DigNum (严格)"("Disabled"=w4298) -> ()  [unwired: 2 in, 2 out]
                n2699 = local read "从板个数"() -> (w4296:dbl)
                n2700 = property on="系统时钟" class="Str"("Disabled"=w4298) -> ()  [unwired: 2 in, 2 out]
                n2701 = property on="配置文件版本" class="Str"("Disabled"=w4298) -> ()  [unwired: 2 in, 2 out]
                n2702 = property on="车架(牌)号" class="Str"("Disabled"=w4298) -> ()  [unwired: 2 in, 2 out]
                n2703 = property on="产品编号" class="Str"("Disabled"=w4298) -> ()  [unwired: 2 in, 2 out]
                n2704 = control-ref of="项目信息"() -> (w4297:refnum<vi>)
                n2705 = stacked-sequence {
                  tunnel: w4297 -> [w4307 w4310]
                  tunnel: w4296 -> [w4306 w4309]
                  frame #0 {
                    n2706 = Compound Arithmetic op=ADD(1.0 ("值"), w4306) -> (w4303:dbl)
                    n2707 = Bundle(w4303, 0) -> (w4305:cluster{dbl, i32})  [unwired: 1 out]
                    n2708 = property class="Tbl (严格)"(reference=w4307, "Index Values"=w4305) -> ()  [unwired: 1 in, 2 out]
                  }
                  frame #1 {
                    n2709 = for {
                      N: 20 -> [_]
                      tunnel: w4310 -> [w4318]
                      tunnel: w4309 -> [w4313]
                      i -> [w4312]
                      n2710 = Compound Arithmetic op=ADD(1.0 ("值"), w4313, w4312) -> (w4315:dbl)
                      n2711 = Bundle(w4315, 0) -> (w4317:cluster{dbl, i32})  [unwired: 1 out]
                      n2712 = property class="Tbl (严格)"(reference=w4318, "Active Cell"=w4317, "Cell BG Color"=u32 6618880) -> ()  [unwired: 1 in, 2 out]
                    }
                  }
                }
                n2713 = Select(t=0, s=w4286, f=1) -> (s? t:f=w4287:i32)
                n2714 = property on="项目信息" class="Tbl (严格)"("Disabled"=w4287) -> ()  [unwired: 2 in, 2 out]
                n2715 = global read "功能码全局.vi" "主板项目信息5"() -> (w4294:bool[])
                n2716 = global read "功能码全局.vi" "主板项目信息6"() -> (w4292:bool[])
                n2717 = Index Array(array=w4294, index=2 ("索引")) -> (element=w4291:bool)
                n2718 = Index Array(array=w4292, index=3 ("索引")) -> (element=w4290:bool)
                n2719 = Not(x=w4300) -> (.not. x?=w4299:bool)
              }
              frame "电压起始值" {
                w4332 = 2
                w4334 = FALSE
                n2720 = property on="从板个数" class="DigNum (严格)"("NumText.BGColor"=u32 13816530) -> ()  [unwired: 2 in, 2 out]
                n2721 = property on="电池实际容量(A)" class="DigNum (严格)"("Disabled"=w4332) -> ()  [unwired: 2 in, 2 out]
                n2722 = property on="使用者" class="DigNum (严格)"("Disabled"=w4332) -> ()  [unwired: 2 in, 2 out]
                n2723 = property on="SOH(%)" class="DigNum (严格)"("Disabled"=w4332) -> ()  [unwired: 2 in, 2 out]
                n2724 = property on="电池额定容量(A)" class="DigNum (严格)"("Disabled"=w4332) -> ()  [unwired: 2 in, 2 out]
                n2725 = property on="SOC(%)" class="DigNum (严格)"("Disabled"=w4332) -> ()  [unwired: 2 in, 2 out]
                n2726 = local read "从板个数"() -> (w4330:dbl)
                n2727 = property on="系统时钟" class="Str"("Disabled"=w4332) -> ()  [unwired: 2 in, 2 out]
                n2728 = property on="配置文件版本" class="Str"("Disabled"=w4332) -> ()  [unwired: 2 in, 2 out]
                n2729 = property on="车架(牌)号" class="Str"("Disabled"=w4332) -> ()  [unwired: 2 in, 2 out]
                n2730 = property on="产品编号" class="Str"("Disabled"=w4332) -> ()  [unwired: 2 in, 2 out]
                n2731 = control-ref of="项目信息"() -> (w4331:refnum<vi>)
                n2732 = stacked-sequence {
                  tunnel: w4331 -> [w4341 w4344 w4357]
                  tunnel: w4330 -> [w4340 w4343 w4356]
                  frame #0 {
                    n2733 = Compound Arithmetic op=ADD(21.0 ("值"), w4340) -> (w4337:dbl)
                    n2734 = Bundle(w4337, 0) -> (w4339:cluster{dbl, i32})  [unwired: 1 out]
                    n2735 = property class="Tbl (严格)"(reference=w4341, "Index Values"=w4339) -> ()  [unwired: 1 in, 2 out]
                  }
                  frame #1 {
                    n2736 = for {
                      N: 10 -> [_]
                      tunnel: w4344 -> [w4354]
                      tunnel: w4343 -> [w4349]
                      i -> [w4348]
                      n2737 = Multiply(x=w4349, y=2.0) -> (x*y=w4346:dbl)
                      n2738 = Compound Arithmetic op=ADD(21.0 ("值"), w4346, w4348) -> (w4351:dbl)
                      n2739 = Bundle(w4351, 0) -> (w4353:cluster{dbl, i32})  [unwired: 1 out]
                      n2740 = property class="Tbl (严格)"(reference=w4354, "Active Cell"=w4353, "Cell BG Color"=u32 16448250) -> ()  [unwired: 1 in, 2 out]
                    }
                  }
                  frame #2 {
                    n2741 = Increment(x=w4356) -> (x+1=w4355:dbl)
                    n2742 = for {
                      N: w4355 -> [_]
                      tunnel: w4357 -> [w4365]
                      tunnel: w4356 -> [w4360]
                      i -> [w4359]
                      n2743 = Compound Arithmetic op=ADD(21.0 ("值"), w4360, w4359) -> (w4362:dbl)
                      n2744 = Bundle(w4362, 0) -> (w4364:cluster{dbl, i32})  [unwired: 1 out]
                      n2745 = property class="Tbl (严格)"(reference=w4365, "Active Cell"=w4364, "Cell BG Color"=u32 6618880) -> ()  [unwired: 1 in, 2 out]
                    }
                  }
                }
                n2746 = Select(t=0, s=w4321, f=1) -> (s? t:f=w4320:i32)
                n2747 = property on="项目信息" class="Tbl (严格)"("Disabled"=w4320) -> ()  [unwired: 2 in, 2 out]
                n2748 = global read "功能码全局.vi" "主板项目信息5"() -> (w4328:bool[])
                n2749 = global read "功能码全局.vi" "主板项目信息6"() -> (w4326:bool[])
                n2750 = Index Array(array=w4328, index=3 ("索引")) -> (element=w4324:bool)
                n2751 = Index Array(array=w4326, index=4 ("索引")) -> (element=w4325:bool)
                n2752 = Not(x=w4334) -> (.not. x?=w4333:bool)
              }
              frame "温度个数" {
                w4379 = 2
                w4381 = FALSE
                n2753 = property on="电池实际容量(A)" class="DigNum (严格)"("Disabled"=w4379) -> ()  [unwired: 2 in, 2 out]
                n2754 = property on="使用者" class="DigNum (严格)"("Disabled"=w4379) -> ()  [unwired: 2 in, 2 out]
                n2755 = property on="SOH(%)" class="DigNum (严格)"("Disabled"=w4379) -> ()  [unwired: 2 in, 2 out]
                n2756 = property on="电池额定容量(A)" class="DigNum (严格)"("Disabled"=w4379) -> ()  [unwired: 2 in, 2 out]
                n2757 = property on="SOC(%)" class="DigNum (严格)"("Disabled"=w4379) -> ()  [unwired: 2 in, 2 out]
                n2758 = local read "从板个数"() -> (w4377:dbl)
                n2759 = control-ref of="项目信息"() -> (w4378:refnum<vi>)
                n2760 = stacked-sequence {
                  tunnel: w4378 -> [w4386 w4389 w4396]
                  tunnel: w4377 -> [w4383 w4388 w4395]
                  frame #0 {
                    n2761 = Bundle("从板个数"=w4383, 0) -> (w4385:cluster{"从板个数":dbl, i32})  [unwired: 1 out]
                    n2762 = property class="Tbl (严格)"(reference=w4386, "Index Values"=w4385) -> ()  [unwired: 1 in, 2 out]
                  }
                  frame #1 {
                    n2763 = for {
                      N: 20 -> [_]
                      tunnel: w4389 -> [w4394]
                      tunnel: w4388 -> [_]
                      i -> [w4390]
                      n2764 = Bundle(w4390, 0) -> (w4393:cluster{i32, i32})  [unwired: 1 out]
                      n2765 = property class="Tbl (严格)"(reference=w4394, "Active Cell"=w4393, "Cell BG Color"=u32 16448250) -> ()  [unwired: 1 in, 2 out]
                    }
                  }
                  frame #2 {
                    n2766 = for {
                      N: w4395 -> [_]
                      tunnel: w4396 -> [w4403]
                      tunnel: w4395 -> [w4397]
                      i -> [w4398]
                      n2767 = Compound Arithmetic op=ADD(w4397, w4398) -> (w4400:dbl)
                      n2768 = Bundle(w4400, 0) -> (w4402:cluster{dbl, i32})  [unwired: 1 out]
                      n2769 = property class="Tbl (严格)"(reference=w4403, "Active Cell"=w4402, "Cell BG Color"=u32 6618880) -> ()  [unwired: 1 in, 2 out]
                    }
                  }
                }
                n2770 = property on="系统时钟" class="Str"("Disabled"=w4379) -> ()  [unwired: 2 in, 2 out]
                n2771 = property on="配置文件版本" class="Str"("Disabled"=w4379) -> ()  [unwired: 2 in, 2 out]
                n2772 = property on="车架(牌)号" class="Str"("Disabled"=w4379) -> ()  [unwired: 2 in, 2 out]
                n2773 = property on="产品编号" class="Str"("Disabled"=w4379) -> ()  [unwired: 2 in, 2 out]
                n2774 = property on="从板个数" class="DigNum (严格)"("NumText.BGColor"=u32 13816530) -> ()  [unwired: 2 in, 2 out]
                n2775 = Select(t=0, s=w4368, f=1) -> (s? t:f=w4367:i32)
                n2776 = property on="项目信息" class="Tbl (严格)"("Disabled"=w4367) -> ()  [unwired: 2 in, 2 out]
                n2777 = global read "功能码全局.vi" "主板项目信息5"() -> (w4375:bool[])
                n2778 = global read "功能码全局.vi" "主板项目信息6"() -> (w4373:bool[])
                n2779 = Index Array(array=w4375, index=4 ("索引")) -> (element=w4371:bool)
                n2780 = Index Array(array=w4373, index=5 ("索引")) -> (element=w4372:bool)
                n2781 = Not(x=w4381) -> (.not. x?=w4380:bool)
              }
              frame "温度起始值" {
                w4417 = 2
                w4419 = FALSE
                n2782 = property on="电池实际容量(A)" class="DigNum (严格)"("Disabled"=w4417) -> ()  [unwired: 2 in, 2 out]
                n2783 = property on="使用者" class="DigNum (严格)"("Disabled"=w4417) -> ()  [unwired: 2 in, 2 out]
                n2784 = property on="SOH(%)" class="DigNum (严格)"("Disabled"=w4417) -> ()  [unwired: 2 in, 2 out]
                n2785 = property on="电池额定容量(A)" class="DigNum (严格)"("Disabled"=w4417) -> ()  [unwired: 2 in, 2 out]
                n2786 = property on="SOC(%)" class="DigNum (严格)"("Disabled"=w4417) -> ()  [unwired: 2 in, 2 out]
                n2787 = local read "从板个数"() -> (w4415:dbl)
                n2788 = property on="系统时钟" class="Str"("Disabled"=w4417) -> ()  [unwired: 2 in, 2 out]
                n2789 = property on="配置文件版本" class="Str"("Disabled"=w4417) -> ()  [unwired: 2 in, 2 out]
                n2790 = property on="车架(牌)号" class="Str"("Disabled"=w4417) -> ()  [unwired: 2 in, 2 out]
                n2791 = property on="产品编号" class="Str"("Disabled"=w4417) -> ()  [unwired: 2 in, 2 out]
                n2792 = control-ref of="项目信息"() -> (w4416:refnum<vi>)
                n2793 = stacked-sequence {
                  tunnel: w4416 -> [w4428 w4431 w4444]
                  tunnel: w4415 -> [w4421 w4430 w4443]
                  frame #0 {
                    n2794 = Multiply(x=w4421, y=3.0) -> (x*y=w4423:dbl)
                    n2795 = Compound Arithmetic op=ADD(23.0 ("值"), w4423) -> (w4425:dbl)
                    n2796 = Bundle(w4425, 0) -> (w4427:cluster{dbl, i32})  [unwired: 1 out]
                    n2797 = property class="Tbl (严格)"(reference=w4428, "Index Values"=w4427) -> ()  [unwired: 1 in, 2 out]
                  }
                  frame #1 {
                    n2798 = for {
                      N: 10 -> [_]
                      tunnel: w4431 -> [w4441]
                      tunnel: w4430 -> [w4436]
                      i -> [w4435]
                      n2799 = Multiply(x=4.0, y=w4436) -> (x*y=w4433:dbl)
                      n2800 = Compound Arithmetic op=ADD(24.0 ("值"), w4433, w4435) -> (w4438:dbl)
                      n2801 = Bundle(w4438, 0) -> (w4440:cluster{dbl, i32})  [unwired: 1 out]
                      n2802 = property class="Tbl (严格)"(reference=w4441, "Active Cell"=w4440, "Cell BG Color"=u32 16448250) -> ()  [unwired: 1 in, 2 out]
                    }
                  }
                  frame #2 {
                    n2803 = Increment(x=w4443) -> (x+1=w4442:dbl)
                    n2804 = for {
                      N: w4442 -> [_]
                      tunnel: w4444 -> [w4454]
                      tunnel: w4443 -> [w4449]
                      i -> [w4448]
                      n2805 = Multiply(x=3.0, y=w4449) -> (x*y=w4446:dbl)
                      n2806 = Compound Arithmetic op=ADD(23.0 ("值"), w4446, w4448) -> (w4451:dbl)
                      n2807 = Bundle(w4451, 0) -> (w4453:cluster{dbl, i32})  [unwired: 1 out]
